vi "Voltage - Continuous Input-.vi"() -> ()   [LabVIEW 2012]
doc: "This example demonstrates how to continuously acquire buffered voltage measurements using a DAQmx device.\n\nFor instructions on how to connect your signals to the DAQ device, refer to your device documentation."
uses:
  <vilib>/DAQmx/read.llb/DAQmx Read (Analog 2D DBL NChan NSamp).vi
  <vilib>/DAQmx/create/channels.llb/DAQmx Create Channel (AI-Voltage-Basic).vi
  <vilib>/DAQmx/configure/timing.llb/DAQmx Timing (Sample Clock).vi
  <vilib>/DAQmx/miscellaneous.llb/DAQmx Fill In Error Info.vi
panel:
  in  "action":i32(ring)=2 items=["verify"=2, "reserve"=4, "commit"=3, "unreserve"=5, "abort"=6]
  out "x-y 3":u32=109
  out "x-y 2":u32=1
  out "x-y":u32=114
  out "Loop time ms":u32=114
  in  "Physical Channel 1":tag="Dev5/ai1"
  out "size(s)":i32[](array[numeric])=[1, 100]
  in  "Stop":bool
  out "Waveform Graph":dbl[][](graph)=[[0.9931523329148897, 0.9931523329148897, 1.0033283036736582, 0.9931523329148897, 0.9931523329148897, 0.9931523329148897, 1.0033283036736582, 0.9931523329148897, 0.9931523329148897, 0.9931523329148897, 0.9931523329148897, 0.9931523329148897, 0.9931523329148897, 0.9931523329148897, 0.9931523329148897, 0.9931523329148897, 0.9931523329148897, 0.9931523329148897, 0.9931523329148897, 0.9931523329148897, 1.0033283036736582, 0.9931523329148897, 0.9931523329148897, 1.0033283036736582, 0.9931523329148897, 0.9931523329148897, 0.9931523329148897, 1.0033283036736582, 0.9931523329148897, 0.9931523329148897, 0.9931523329148897, 0.9931523329148897, 1.0033283036736582, 0.9931523329148897, 1.0033283036736582, 0.9931523329148897, 0.9931523329148897, 1.0033283036736582, 0.9931523329148897, 0.9931523329148897, 0.9931523329148897, 0.9931523329148897, 0.9931523329148897, 0.9931523329148897, 0.9931523329148897, 0.9931523329148897, 0.9931523329148897, 1.0033283036736582, 1.0033283036736582, 0.9931523329148897, 0.9931523329148897, 0.9931523329148897, 1.0033283036736582, 0.9931523329148897, 0.9931523329148897, 0.9931523329148897, 0.9931523329148897, 0.9931523329148897, 0.9931523329148897, 1.0033283036736582, 0.9931523329148897, 0.9931523329148897, 0.9931523329148897, 0.9931523329148897, 0.9931523329148897, 0.9931523329148897, 1.0033283036736582, 0.9931523329148897, 0.9931523329148897, 0.9931523329148897, 0.9931523329148897, 0.9931523329148897, 1.0033283036736582, 1.0033283036736582, 1.0033283036736582, 0.9931523329148897, 0.9931523329148897, 0.9931523329148897, 0.9931523329148897, 0.9931523329148897, 0.9931523329148897, 0.9931523329148897, 0.9931523329148897, 0.9931523329148897, 0.9931523329148897, 0.9931523329148897, 1.0033283036736582, 1.0033283036736582, 0.9931523329148897, 0.9931523329148897, 0.9931523329148897, 0.9931523329148897, 0.9931523329148897, 1.0033283036736582, 0.9931523329148897, 0.9931523329148897, 0.9931523329148897, 1.0033283036736582, 0.9931523329148897, 0.9931523329148897]]
  in  "Samples per Loop":i32=100
  in  "Sample Rate":dbl=1000.0
  in  "Sample Clock Source":tag="OnboardClock"
  in  "Terminal Configuration":i32(ring)=10083 items=["default"=-1, "RSE"=10083, "NRSE"=10078, "Differential"=10106, "Pseudodifferential"=12529]
  in  "Max Voltage":dbl=5.0
  in  "Min Voltage":dbl
  in  "Physical Channel 0":tag="Dev5/ai0"
  # "Channel Settings"
  # "Acquired Data"
  # "Timing Settings"
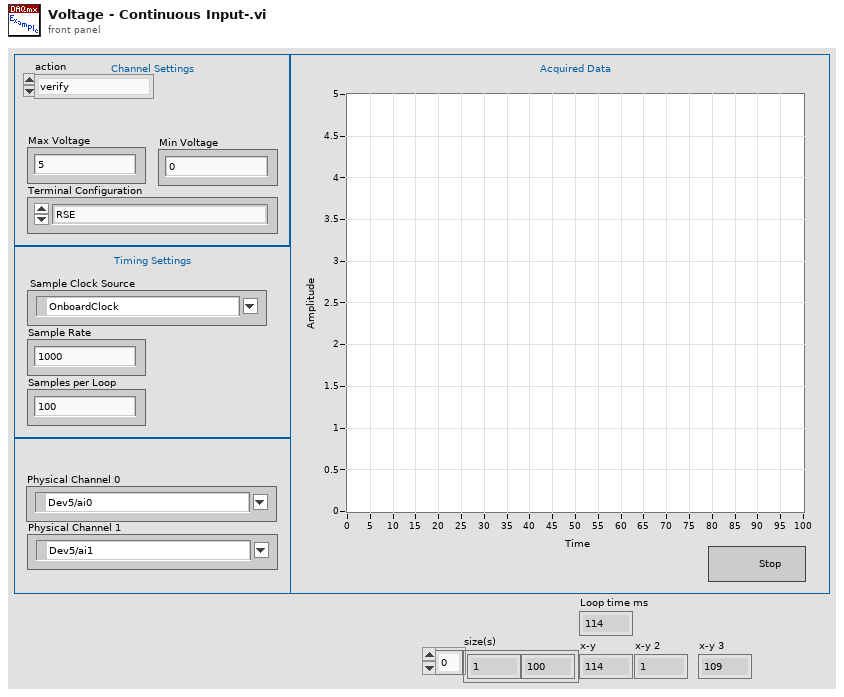
[diagram p1: front panel]
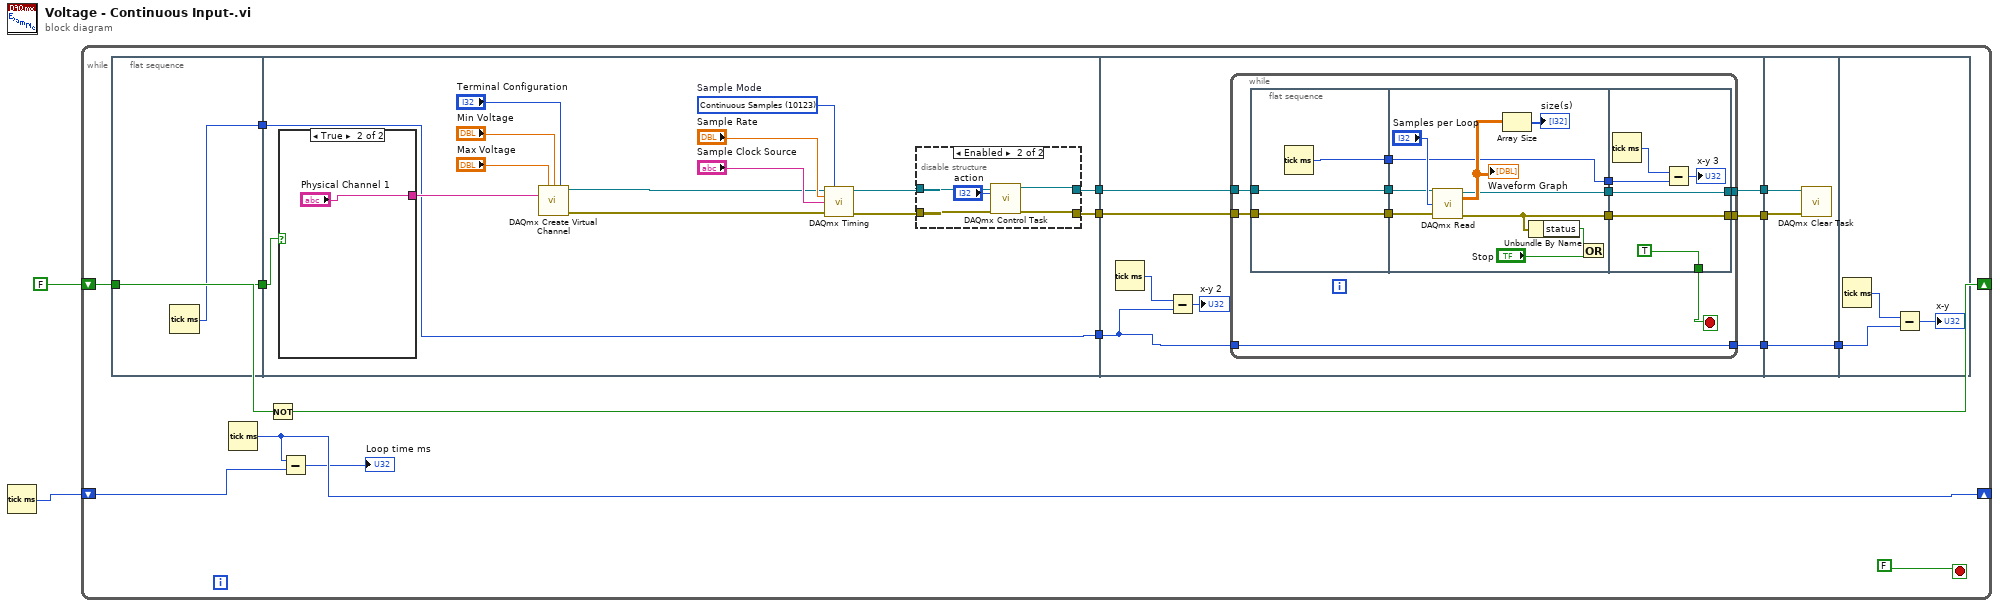
[diagram p0: block diagram]
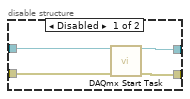
[diagram p2: hidden frame]
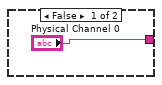
[diagram p3: hidden frame]
diagram:
  n1 = Tick Count (ms)() -> (millisecond timer value=w1:u32)
  n2 = while {
    shift-right: [w16] -> _
    shift-left: FALSE -> [w12]
    shift-right: [w14] -> _
    shift-left: w1 -> [w15]
    stop <- FALSE stop-if-true
    n3 = flat-sequence {
      tunnel: w12 -> [w19]
      tunnel: [w19] -> w8
      tunnel: [w18] -> w7
      tunnel: [w22] -> w11
      tunnel: [w21] -> w10
      tunnel: [w20] -> w9
      tunnel: w8 -> [w23]
      tunnel: w7 -> [w20]
      tunnel: w11 -> [w53]
      tunnel: w10 -> [w52]
      tunnel: w9 -> [w46]
      tunnel: [w51] -> w6
      tunnel: [w50] -> w5
      tunnel: [w48] -> w4
      tunnel: w6 -> [w86]
      tunnel: w5 -> [w85]
      tunnel: w4 -> [w87]
      tunnel: [w87] -> w3
      tunnel: w3 -> [w88]
      frame #0 {
        n4 = Tick Count (ms)() -> (millisecond timer value=w18:u32)
      }
      frame #1 {
        w34 = 10123 items=["Finite Samples"=10178, "Continuous Samples"=10123, "Hardware Timed Single Point"=12522]  # Sample Mode
        n5 = case shown="True" w23 {
          tunnel: ["Physical Channel 0" "Physical Channel 1"] -> w24
          frame False {
          }
          frame True {
          }
        }
        n6 = call-poly <vilib>:"DAQmx Create Virtual Channel.vi"("maximum value"="Max Voltage", "minimum value"="Min Voltage", "input terminal configuration"="Terminal Configuration", "physical channels"=w24) -> ("task out"=w26:refnum<k21>, "error out"=w25:errorcluster)  [unwired: 10 in]
        n7 = call-poly <vilib>:"DAQmx Timing.vi"("task/channels in"=w26, "sample mode"=w34, "rate"="Sample Rate", "source"="Sample Clock Source", "error in"=w25) -> ("task out"=w28:refnum<k21>, "error out"=w27:errorcluster)  [unwired: 9 in]
        n8 = disable-structure shown="Enabled" {
          disable-tunnel: w28 -> [w38 w43]
          disable-tunnel: w27 -> [w37 w42]
          disable-tunnel: [w36 w41] -> w22
          disable-tunnel: [w35 w40] -> w21
          frame Disabled {
            n9 = call <vilib>:"DAQmx Start Task.vi"("task/channels in"=w38, "error in"=w37) -> ("task out"=w36:refnum<k21>, "error out"=w35:errorcluster)  [unwired: 12 in]
          }
          frame Enabled {
            n10 = call <vilib>:"DAQmx Control Task.vi"("task/channels in"=w43, "action"="action", "error in"=w42) -> ("task out"=w41:refnum<k21>, "error out"=w40:errorcluster)  [unwired: 11 in]
          }
        }
      }
      frame #2 {
        n11 = Tick Count (ms)() -> (millisecond timer value=w47:u32)
        n12 = Subtract(x=w47, y=w46) -> (x-y=→"x-y 2":u32)
        n13 = while {
          tunnel: [w61] -> w51
          tunnel: [w62] -> w50
          tunnel: w53 -> [w65]
          tunnel: w52 -> [w64]
          tunnel: [w63] -> w48
          tunnel: w46 -> [w63]
          stop <- w54 stop-if-true
          n14 = flat-sequence {
            tunnel: w64 -> [w67]
            tunnel: w65 -> [w68]
            tunnel: [w68] -> w58
            tunnel: [w67] -> w57
            tunnel: [w66] -> w55
            tunnel: [w71] -> w60
            tunnel: [w70] -> w59
            tunnel: w58 -> [w74]
            tunnel: w57 -> [w73]
            tunnel: [w69] -> w56
            tunnel: w55 -> [w69]
            tunnel: [w83] -> w61
            tunnel: [w84] -> w62
            tunnel: w60 -> [w84]
            tunnel: w59 -> [w83]
            tunnel: w56 -> [w80]
            tunnel: [TRUE] -> w54
            frame #0 {
              n15 = Tick Count (ms)() -> (millisecond timer value=w66:u32)
            }
            frame #1 {
              n16 = call-poly <vilib>:"DAQmx Read.vi"("task/channels in"=w74, "number of samples per channel"="Samples per Loop", "error in"=w73) -> ("task out"=w70:refnum<k21>, "data"=w72:dbl[][], "error out"=w71:errorcluster)  [unwired: 10 in]
              "Waveform Graph" <- w72
              n17 = Array Size(array=w72) -> (size(s)=→"size(s)":i32[])
              n18 = Unbundle By Name(w71) -> ("status"=w78:bool)
              n19 = Or(x=w78, y="Stop") -> ()  [unwired: 1 out]
            }
            frame #2 {
              n20 = Tick Count (ms)() -> (millisecond timer value=w81:u32)
              n21 = Subtract(x=w81, y=w80) -> (x-y=→"x-y 3":u32)
            }
          }
        }
      }
      frame #3 {
        n22 = call <vilib>:"DAQmx Clear Task.vi"("task in"=w86, "error in"=w85) -> ()  [unwired: 13 in, 1 out]
      }
      frame #4 {
        n23 = Tick Count (ms)() -> (millisecond timer value=w89:u32)
        n24 = Subtract(x=w89, y=w88) -> (x-y=→"x-y":u32)
      }
    }
    n25 = Tick Count (ms)() -> (millisecond timer value=w14:u32)
    n26 = Not(x=w12) -> (.not. x?=w16:bool)
    n27 = Subtract(x=w14, y=w15) -> (x-y=→"Loop time ms":u32)
  }
